vi "01 Cambios de fase.vi"() -> ()   [LabVIEW 2021]
panel:
  out "Exotérmico":bool
  out "Endotérmico":bool
  out "Calor Latente":dbl(knob) scale=-1000.0..1000.0
  in  "Masa (g)":dbl caption="Masa"
  in  "Proceso":dbl(ring)=40.7 items=["Evaporación"=40.7, "Solidificación"=-6.02, "Deposición"=-46.72, "Sublimación"=46.72, "Fusion "=6.02, "Condensación"=-40.7]
  in  "stop":bool
  # "CAMBIOS DE FASE - AGUA"
  # "Desarrollado por:\n     Semillero Electroquimica e Innovación Ambiental - SEIA"
  # "Calor Latente"
  # "kJ"
  # "g"
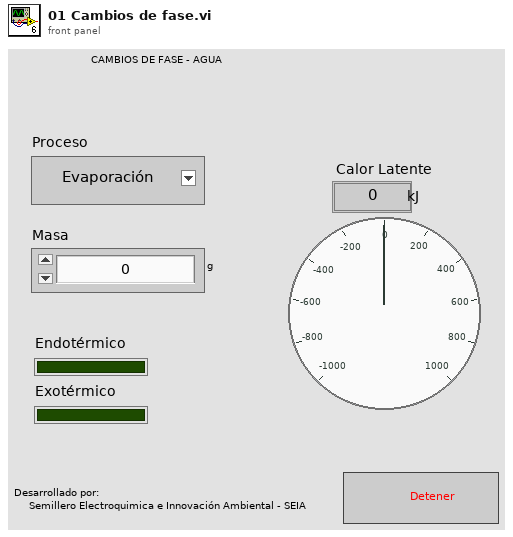
[diagram p1: front panel]
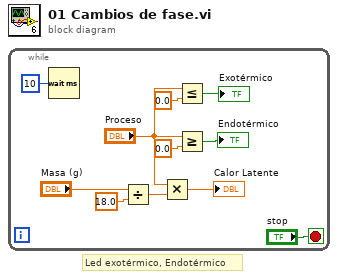
[diagram p0: block diagram]
diagram:
  # "Led exotérmico, Endotérmico"
  n1 = while {
    stop <- "stop" stop-if-true
    n2 = Wait (ms)(milliseconds to wait=u32 10) -> ()  [unwired: 1 out]
    n3 = Divide(x="Masa (g)", y=18.0) -> (x/y=w9:dbl)
    n4 = Multiply(x="Proceso", y=w9) -> (x*y=→"Calor Latente":dbl)
    n5 = Less Or Equal?(x="Proceso", y=0.0) -> (x <= y?=→"Exotérmico":bool)
    n6 = Greater Or Equal?(x="Proceso", y=0.0) -> (x >= y?=→"Endotérmico":bool)
  }
